vi "FreqStep-Tone.vi"(0 "F0 (Hz)":dbl=1000.0, 5 "Fend (Hz)":dbl=2000.0, 7 "Fs (Hz)":dbl=100000.0, 9 "Npts":i32, 11 "Gate Control":T1(xcontrol)) -> (8 "Array":dbl[](array[numeric]), 10 "Omega(t)":dbl[](array[numeric]), 15 "Finst":dbl[](array[numeric]))   [LabVIEW 2015]
uses:
  Controls/Gate XCtl/Gate Control.xctl
panel:
  in  "phase":dbl
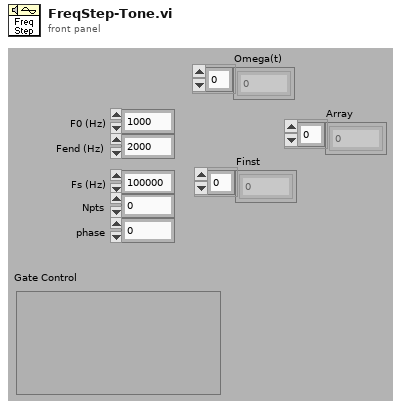
[diagram p1: front panel]
types:
  T1 = cluster{"Active":bool, "Delay (ms)":dbl, "Width (ms)":dbl, "Ramp (ms)":dbl}
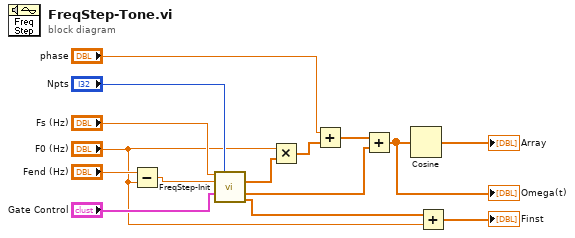
[diagram p0: block diagram]
diagram:
  n1 = Subtract(x="Fend (Hz)", y="F0 (Hz)") -> (x-y=w14:dbl)
  n2 = call "FreqStep-Init.vi"("Fs (Hz)"="Fs (Hz)", "Npts"="Npts", "delta f (Hz)"=w14, "Gate Control"="Gate Control") -> ("omega_1"=w12:dbl[], "omega_2"=w13:dbl[], "delta Finst"=w3:dbl[])  [unwired: 9 in]
  n3 = Multiply(x="F0 (Hz)", y=w12) -> (x*y=w11:dbl[])
  n4 = Add(x="phase", y=w11) -> (x+y=w10:dbl[])
  n5 = Add(x=w10, y=w13) -> (x+y=w9:dbl[])
  "Omega(t)" <- w9
  n6 = Cosine(x=w9) -> (cos(x)=→"Array":dbl[])
  n7 = Add(x=w3, y="F0 (Hz)") -> (x+y=→"Finst":dbl[])
